vi "test Read File.vi"(8 "error in (no error)":errorcluster, 11 "TestCase in":refnum<class "WriteFileTests.lvclass">) -> (0 "error out":errorcluster, 3 "TestCase out":refnum<class "WriteFileTests.lvclass">)   [LabVIEW 2014, in "WriteFileTests.lvclass"]
uses:
  WriteFileTests.lvclass
  <vilib>/addons/_JKI Toolkits/VI Tester/TestCase.llb/TestCase.lvclass
  SPLAT/Position.lvclass
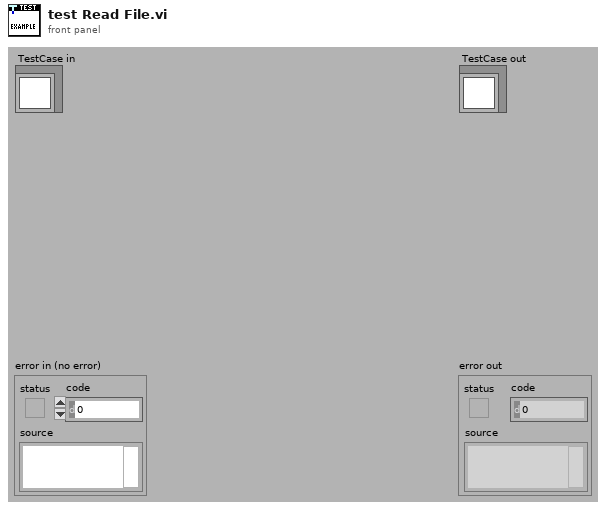
[diagram p1: front panel]
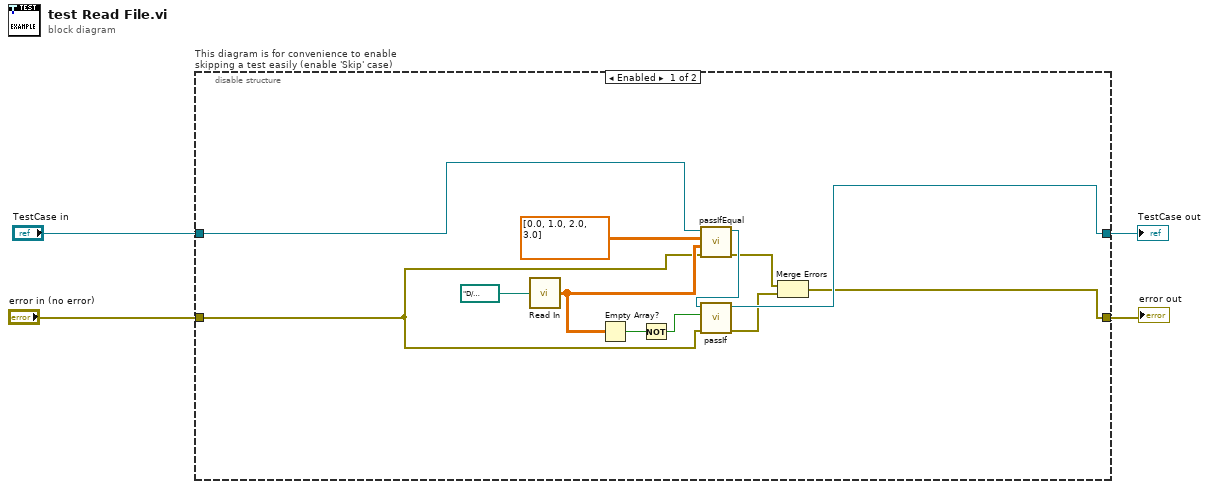
[diagram p0: block diagram]
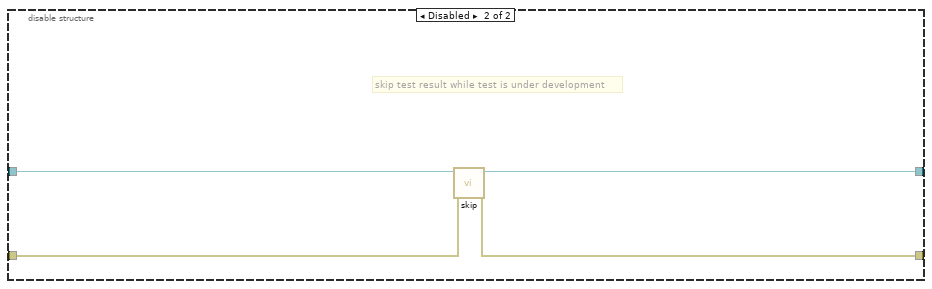
[diagram p2: hidden frame]
diagram:
  n1 = disable-structure "This diagram is for convenience to enable skipping a test easily (enable 'Skip' case)" shown="Enabled" {
    disable-tunnel: "TestCase in" -> [w11 w20]
    disable-tunnel: [w9 w18] -> w1
    disable-tunnel: [w5 w19] -> w3
    disable-tunnel: "error in (no error)" -> [w8 w17]
    frame Enabled {
      n2 = call "Read In.vi"("File path"=path "D:/SPLAT-tests/Write File Test/WriteFileTests/write_data_to_file_testfile.txt") -> ("DataOut [tagID, anchorID, distance, time]"=w13:dbl[][])  [unwired: 14 in]
      n3 = Empty Array?(array=w13) -> (empty?=w15:bool)
      n4 = Not(x=w15) -> (.not. x?=w14:bool)
      n5 = call-dynamic "passIfEqual.vi"("error in (no error)"=w8, "y"=w13, "x"=dbl[][] [[0.0, 1.0, 2.0, 3.0]] ("Array"), "TestCase in"=w11) -> ("error out"=w7:errorcluster, "TestCase out"=w10:refnum<class "WriteFileTests.lvclass">)  [unwired: 6 in]
      n6 = call-dynamic "passIf.vi"("error in (no error)"=w8, "pass"=w14, "TestCase in"=w10) -> ("error out"=w6:errorcluster, "TestCase out"=w9:refnum<class "WriteFileTests.lvclass">)  [unwired: 7 in]
      n7 = Merge Errors(w7, w6) -> (w5:errorcluster)
    }
    frame Disabled {
      # "skip test result while test is under development"
      n8 = call <vilib>:"skip.vi"("error in (no error)"=w17, "TestCase in"=w20) -> ("error out"=w19:errorcluster, "TestCase out"=w18:refnum<class "WriteFileTests.lvclass">)  [unwired: 8 in]
    }
  }
  "error out" <- w3
  "TestCase out" <- w1
